vi "PotValueToDegrees.vi"(0 "PotIn":dbl) -> (2 "Degrees":dbl)   [LabVIEW 2015]
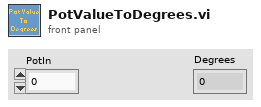
[diagram p1: front panel]
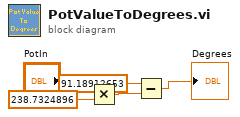
[diagram p0: block diagram]
diagram:
  n1 = Multiply(x="PotIn", y=238.7324896) -> (x*y=w3:dbl)
  n2 = Subtract(x=91.18912653, y=w3) -> (x-y=→"Degrees":dbl)
